vi "PIXY Object Handler.vi"(10 "Normal Object":bool, 11 "Accumulated Words":u8[](array[numeric]) format="%.0x") -> (0 "Angle":i16, 1 "CheckSum Error":bool, 2 "Valid":bool, 3 "Object":T1)   [LabVIEW 2016]
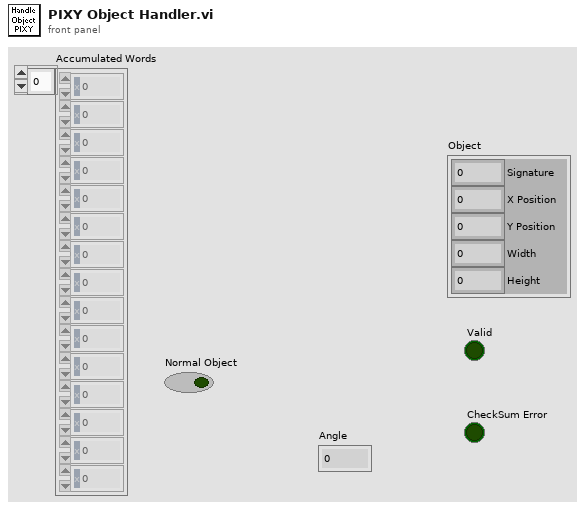
[diagram p1: front panel]
types:
  T1 = cluster{"Signature":u16, "X Position":u16, "Y Position":u16, "Width":u16, "Height":u16}
  T2 = cluster{"Num to Read":u16, "Num to Read":u16, "Num to Read":u16, "Num to Read":u16, "Num to Read":u16}
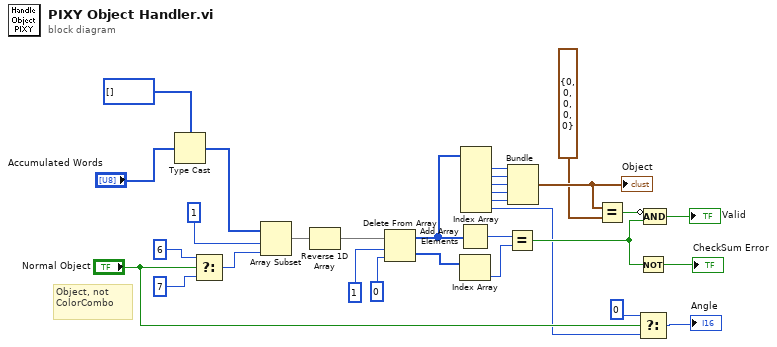
[diagram p0: block diagram]
diagram:
  # "Object, not\nColorCombo"
  n1 = Type Cast(type=u16[] [], x="Accumulated Words") -> (*(type *) &x=w1:u16[])
  n2 = Select(t=6 ("Num to Read"), s="Normal Object", f=7 ("Num to Read")) -> (s? t:f=w8:i32)
  n3 = Array Subset(array=w1, index=1 ("Num to Read"), length=w8) -> (w18:u16[])
  n4 = Reverse 1D Array(array=w18) -> (reversed array=w19:u16[])
  n5 = Delete From Array(array=w19, length=1 ("Num to Read"), index=0 ("Num to Read")) -> (deleted portion=w23:u16[], array with subset deleted=w25:u16[])
  n6 = Add Array Elements(numeric array=w25) -> (sum=w22:u16)
  n7 = Index Array(array=w23) -> (element=w24:u16)  [unwired: 1 in]
  n8 = Index Array(array=w25) -> (element #1=w30:u16, element #2=w29:u16, element #3=w28:u16, element #4=w27:u16, element #5=w26:u16, element #6=w4:u16)  [unwired: 6 in]
  n9 = Equal?(x=w22, y=w24) -> (x = y?=w10:bool)
  n10 = Bundle("Num to Read"=w30, "Num to Read"=w29, "Num to Read"=w28, "Num to Read"=w27, "Num to Read"=w26) -> (w15:T2)  [unwired: 1 in]
  "Object" <- w15
  n11 = Equal?(x=w15, y=T1 {"Signature"=0, "X Position"=0, "Y Position"=0, "Width"=0, "Height"=0} ("Object")) -> (x = y?=w13:bool)
  n12 = Not(x=w10) -> (.not. x?=→"CheckSum Error":bool)
  n13 = Select(t=u16 0 ("Num to Read"), s="Normal Object", f=w4) -> (s? t:f=→"Angle":u16)
  n14 = Compound Arithmetic op=AND(invert w13, w10) -> (→"Valid":bool)
